vi "SRAM_Initialized_v1.vi"(11 "ControlBoard VISA":refnum<visa-resource-name>="ControlBoard") -> (2 "Passed?":string, 3 "Test Result":string)   [LabVIEW 2019]
uses:
  <vilib>/Instr/_visa.llb/VISA Flush IO Buffer Mask.ctl
panel:
  out "error out":errorcluster
  in  "error in (no error)":errorcluster
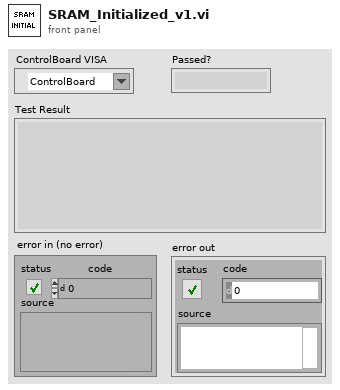
[diagram p1: front panel]
types:
  T1 = typedef "VISA Flush IO Buffer Mask.ctl" = u16
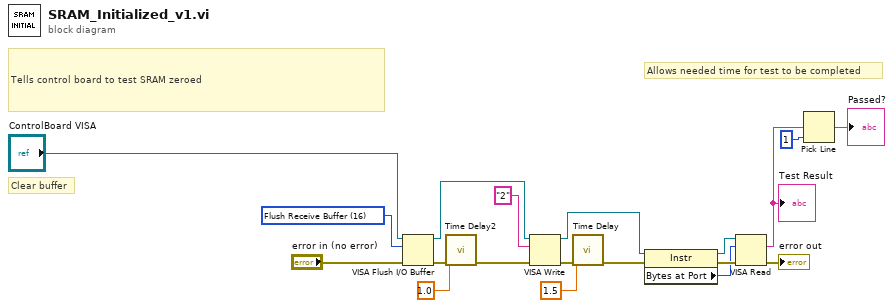
[diagram p0: block diagram]
diagram:
  w18 = T1 16 items=["Flush Receive Buffer"=16, "Write Transmit Buffer to Device"=32, "Flush Receive Buffer (No I/O)"=64, "Flush Transmit Buffer"=128] ("Mask")
  # "Allows needed time for test to be completed"
  # "Tells control board to test SRAM zeroed"
  # "Clear buffer"
  n1 = VISA Flush I/O Buffer(VISA resource name="ControlBoard VISA", mask (16)=w18, error in (no error)="error in (no error)") -> (VISA resource name out=w16:refnum<visa-resource-name>, error out=w13:errorcluster)
  n2 = call "Time Delay2"("error in (no error)"=w13, "Delay Time (s)"=1.0) -> ("error out"=w12:errorcluster)  [unwired: 9 in]
  n3 = VISA Write(VISA resource name=w16, write buffer="2", error in (no error)=w12) -> (VISA resource name out=w10:refnum<visa-resource-name>, error out=w17:errorcluster)  [unwired: 1 out]
  n4 = call "Time Delay"("error in (no error)"=w17, "Delay Time (s)"=1.5) -> ("error out"=w11:errorcluster)  [unwired: 9 in]
  n5 = property class="Instr"(reference=w10, error in=w11) -> (reference out=w9:refnum<visa-resource-name>, error out=w8:errorcluster, "Bytes at Port"=w7:u32)
  n6 = VISA Read(VISA resource name=w9, byte count=w7, error in (no error)=w8) -> (read buffer=w5:string, error out=→"error out":errorcluster)  [unwired: 2 out]
  "Test Result" <- w5
  n7 = Pick Line(multi-line string=w5, line index=1) -> (output string=→"Passed?":string)  [unwired: 1 in]
